vi "fgv_inrange-lidar-data_check.vi"(8 "error in":errorcluster) -> (0 "error out":errorcluster)   [LabVIEW 2019]
uses:
  Ctrl/tim571-databuf.ctl
panel:
  out "XY Graph":T1(graph)
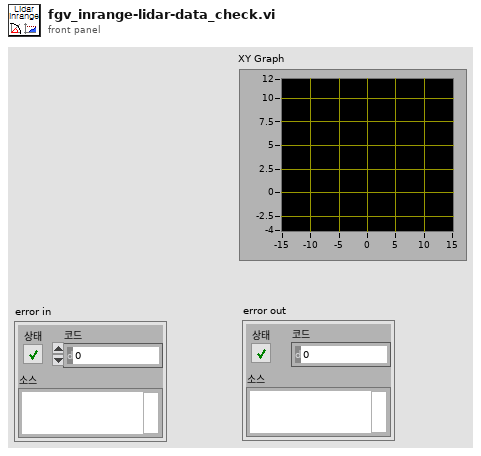
[diagram p1: front panel]
types:
  T1 = cluster{"Array out":cluster{"x":dbl, "y":dbl}[]}[]
  T2 = typedef "tim571-databuf.ctl" = enum16{"write raw data", "write xyz data", "read"}
  T3 = enum16{"none", "VLP16", "TIM571", "RPLidar A2", "RPLidar A3"}
  T4 = typedef "system_hw.ctl" = cluster{"AGV":enum16{"none", "ERP42", "ERP42mini", "Scout", "Ycar"}, "Lidar 1":enum16{"none", "VLP16", "TIM571", "RPLidar A2", "RPLidar A3"}, "Lidar 2":enum16{"none", "VLP16", "TIM571", "RPLidar A2", "RPLidar A3"}, "GPS":enum16{"none", "F9P", "M8P", "PwrPak7", "19X HVS"}, "Camera":enum16{"none", "C920", "C922", "GT1290C", "MS LifeCam"}, "Joystick":enum16{"none", "joystick"}, "sound":enum16{"none", "speaker"}}
  T5 = cluster{"limit inrange xydata":cluster{"x":dbl, "y":dbl}[]}[]
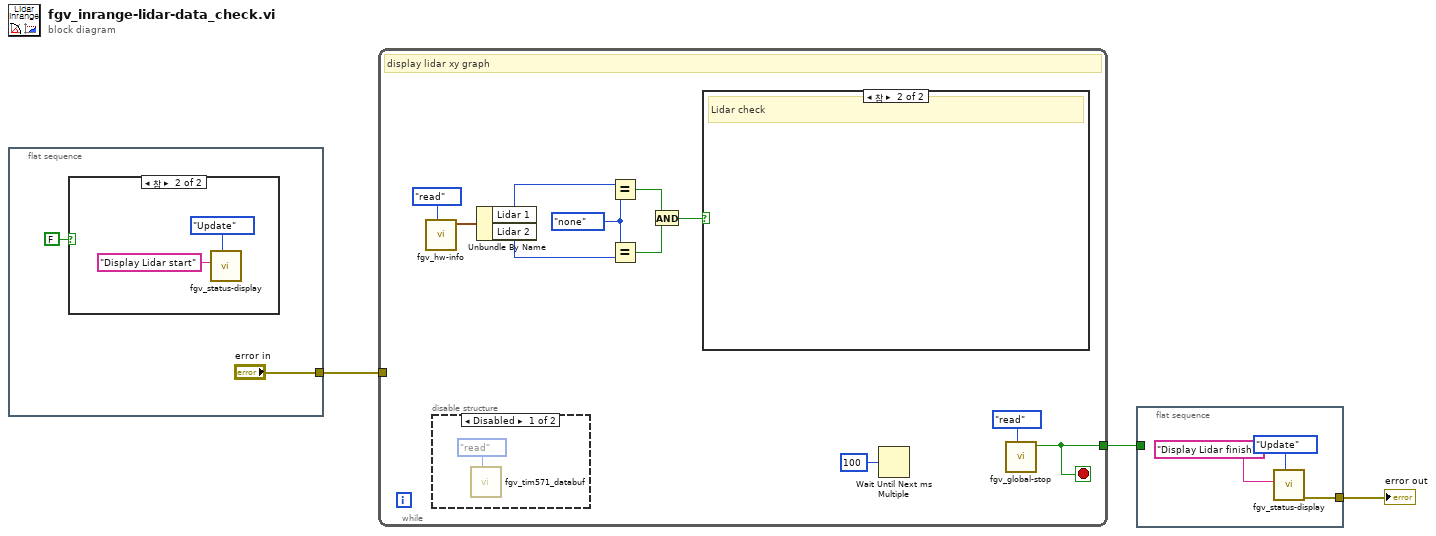
[diagram p0: block diagram]
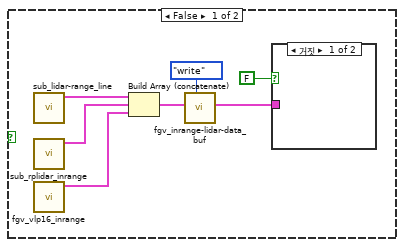
[diagram p3: hidden frame]
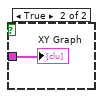
[diagram p4: hidden frame]
diagram:
  n1 = flat-sequence {
    tunnel: ["error in"] -> w1
    frame #0 {
      n2 = case shown="참" FALSE {
        frame False {
        }
        frame True {
          n3 = call "fgv_status-display.vi"("Mode"=enum16{"Initial", "Update", "Clear"}."Update", "title"="Display Lidar start" ("String in 1")) -> ()  [unwired: 9 in, 1 out]
        }
      }
    }
  }
  n4 = while {
    tunnel: [w16] -> w2
    tunnel: w1 -> [_]
    stop <- w16 stop-if-true
    w12 = T3."none" ("y")
    # "display lidar xy graph"
    n5 = call "fgv_hw-info.vi"("cmd"=enum16{"write", "read"}."read") -> ("HW info out"=w14:T4)  [unwired: 10 in]
    n6 = disable-structure shown="Disabled" {
      frame Disabled {
        n7 = call "fgv_tim571_databuf.vi"("cmd"=tim571-databuf."read") -> ()  [unwired: 8 in, 3 out]
      }
      frame Enabled {
      }
    }
    n8 = Unbundle By Name(w14) -> ("Lidar 1"=w13:T3, "Lidar 2"=w11:T3)
    n9 = Equal?(x=w13, y=w12) -> (x = y?=w10:bool)
    n10 = Equal?(x=w12, y=w11) -> (x = y?=w9:bool)
    n11 = And(x=w10, y=w9) -> (x .and. y?=w8:bool)
    n12 = case shown="참" w8 {
      frame False {
        n13 = call "sub_lidar-range_line.vi"() -> ("guide line"=w22:cluster{cluster{"x":dbl, "y":dbl}[]})  [unwired: 11 in]
        n14 = call "sub_rplidar_inrange.vi"() -> ("XY Graph"=w23:T1)  [unwired: 10 in, 1 out]
        n15 = call "fgv_vlp16_inrange.vi"() -> ("data"=w21:T5)  [unwired: 10 in, 1 out]
        n16 = Build Array (concatenate)(w22, w23, w21) -> (w20:T5)
        n17 = call "fgv_inrange-lidar-data_buf.vi"("cmd"=enum16{"read", "write"}."write", "in range data new"=w20) -> ("in range data new out"=w19:T1)  [unwired: 8 in, 1 out]
        n18 = case shown="거짓" FALSE {
          tunnel: w19 -> [_ w26]
          frame False {
          }
          frame True {
            "XY Graph" <- w26
          }
        }
      }
      frame True {
        # "Lidar check"
      }
    }
    n19 = Wait Until Next ms Multiple(millisecond multiple=u32 100 ("milliseconds to wait")) -> ()  [unwired: 1 out]
    n20 = call "fgv_global-stop.vi"("cmd"=enum16{"init", "stop", "read"}."read") -> ("val_out"=w16:bool)  [unwired: 10 in]
  }
  n21 = flat-sequence {
    tunnel: w2 -> [_]
    tunnel: [w28] -> w3
    frame #0 {
      n22 = call "fgv_status-display.vi"("Mode"=enum16{"Initial", "Update", "Clear"}."Update", "title"="Display Lidar finish" ("String in 1")) -> ("error out"=w28:errorcluster)  [unwired: 9 in]
    }
  }
  "error out" <- w3
